vi "Symmetrize (single).vi"(8 "error in (no error)":errorcluster, 11 "XY-data":cluster{"X-array":dbl[], "Y-array":dbl[]} {"Y-array" format="%.2p"; "X-array" format="%.2p"}) -> (0 "error out":errorcluster, 1 "Antisymmetric":cluster{"X-array":dbl[], dbl[]}, 2 "Symmetric":cluster{"X-array":dbl[], dbl[]}, 3 "XY-data out":cluster{"X-array":dbl[], "Y-array":dbl[]} {"Y-array" format="%.2p"; "X-array" format="%.2p"})   [LabVIEW 2019, in "xy_utilities.lvlib"]
doc: "Compute the Symmetric and Antisymmetric functions of <b>XY-data</b>\n\n<b>Symmetric</b>: f+ = (f(x) + f(-x))/2\n<b>Antisymmetric</b>: f- = (f(x) - f(-x))/2"
uses:
  xy_utilities.lvlib
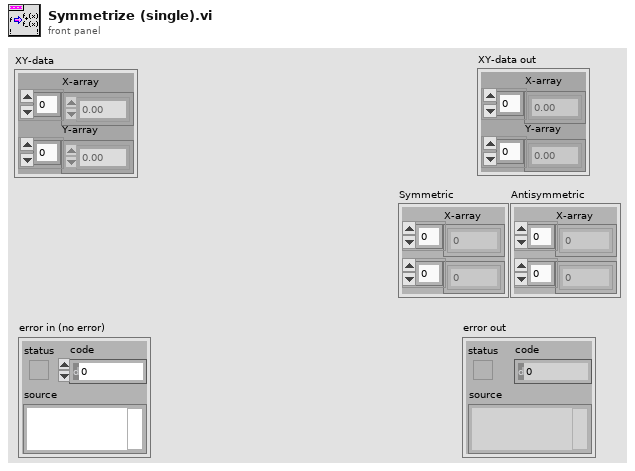
[diagram p1: front panel]
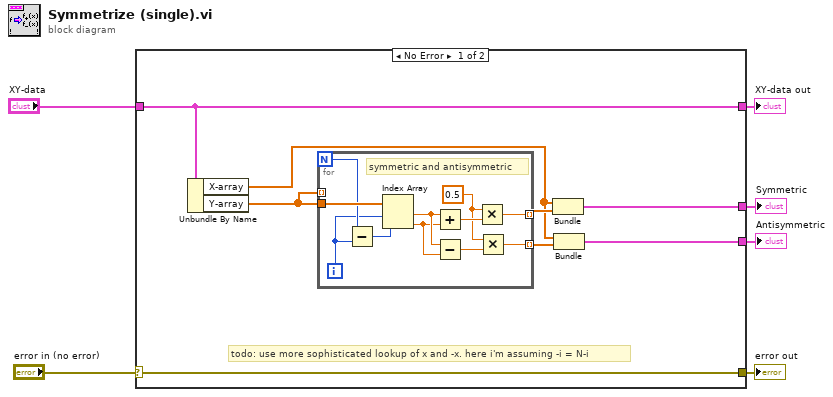
[diagram p0: block diagram]
diagram:
  n1 = case shown="No Error" "error in (no error)" {
    selector: "error in (no error)" -> [w14 w27]
    tunnel: [w14 w27] -> w5
    tunnel: "XY-data" -> [w13 w26]
    tunnel: [w13 w26] -> w3
    tunnel: [w8 _] -> w2
    tunnel: [w7 _] -> w1
    frame No Error {
      # "todo: use more sophisticated lookup of x and -x. here i'm assuming -i = N-i"
      n2 = Unbundle By Name(w13) -> ("X-array"=w9:dbl[], "Y-array"=w10:dbl[])
      n3 = for {
        N -> [w24]
        tunnel: w10 -> [w25]
        tunnel: w10 -> [_] mode=indexing
        tunnel: [w16] -> w11 mode=indexing
        tunnel: [w15] -> w12 mode=indexing
        i -> [w23]
        w17 = 0.5 ("x")
        # "symmetric and antisymmetric"
        n4 = Subtract(x=w24, y=w23) -> (x-y=w22:i32)
        n5 = Index Array(array=w25, index #1=w23, index #2=w22) -> (element #1=w21:dbl, element #2=w20:dbl)
        n6 = Add(x=w21, y=w20) -> (x+y=w19:dbl)
        n7 = Subtract(x=w21, y=w20) -> (x-y=w18:dbl)
        n8 = Multiply(x=w17, y=w19) -> (x*y=w16:dbl)
        n9 = Multiply(x=w17, y=w18) -> (x*y=w15:dbl)
      }
      n10 = Bundle("X-array"=w9, w11) -> (w8:cluster{"X-array":dbl[], dbl[]})  [unwired: 1 in]
      n11 = Bundle("X-array"=w9, w12) -> (w7:cluster{"X-array":dbl[], dbl[]})  [unwired: 1 in]
    }
    frame Error {
    }
  }
  "error out" <- w5
  "XY-data out" <- w3
  "Symmetric" <- w2
  "Antisymmetric" <- w1
